vi "SHARP_2Y0A21_(SubVI).vi"(10 "Stop":bool, 11 "Calibration Parameters":cluster{"m":dbl, "b":dbl, "k":dbl, "c":dbl}={"m"=1.8233599662780762, "b"=0.2962961196899414, "k"=0.17500019073486328, "c"=0.17500019073486328}) -> (0 "error out":errorcluster, 2 "Gauge":dbl(knob) scale=10.0..150.0, 3 "Distance Waveform":dbl(graph))   [LabVIEW 2016]
uses:
  <vilib>/myRIO/Instrument Drivers/Onboard IO/AI/vis/Read.vi
  <vilib>/myRIO/Common/Instrument Driver Framework/myRIO v1.0/UART/vis/myRIO v1.0 Close UART.vi
  <vilib>/myRIO/Instrument Drivers/Onboard IO/AI/vis/Smart Open.vi
  <vilib>/Utility/error.llb/Error Cluster From Error Code.vi
  <vilib>/myRIO/Common/Instrument Driver Framework/myRIO v1.0/AI/vis/myRIO v1.0 Read AI.vi
  <vilib>/myRIO/Common/Instrument Driver Framework/Utilities/vis/FPGA Ref Manager.vi
  <vilib>/myRIO/Common/Instrument Driver Framework/myRIO v1.0/myRIO v1.0 Reset FPGA.vi
  <vilib>/myRIO/Common/Instrument Driver Framework/myRIO v1.0/IRQ/vis/myRIO v1.0 IRQ Info FGV.vi
  <vilib>/myRIO/Common/Instrument Driver Framework/myRIO v1.0/IRQ/vis/myRIO v1.0 Timer IRQ Info FGV.vi
  <vilib>/myRIO/Common/Instrument Driver Framework/myRIO v1.0/IRQ/vis/myRIO v1.0 ISR Agent.vi
  <vilib>/myRIO/Instrument Drivers/Utilities/Utilities.lvlib
panel:
  out "Numeric":dbl
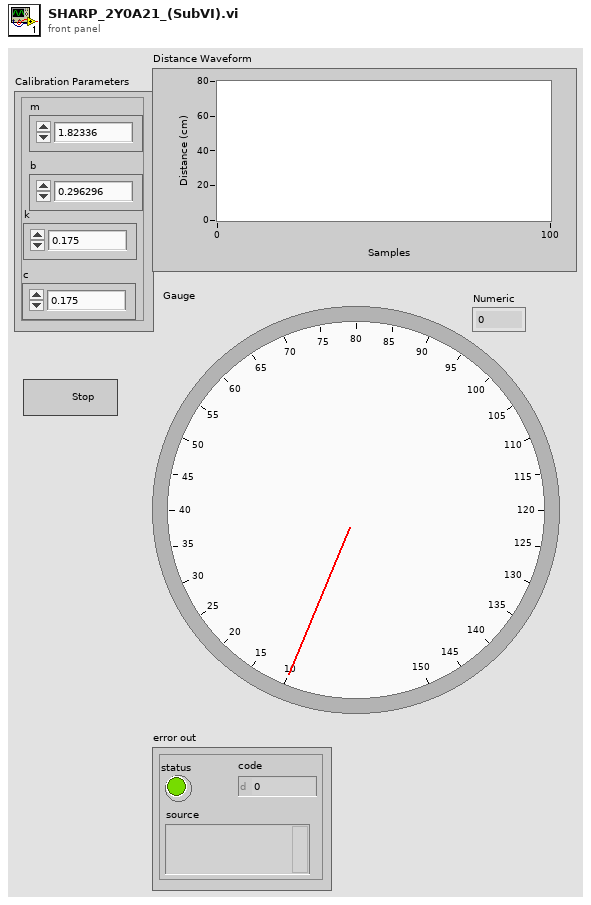
[diagram p1: front panel]
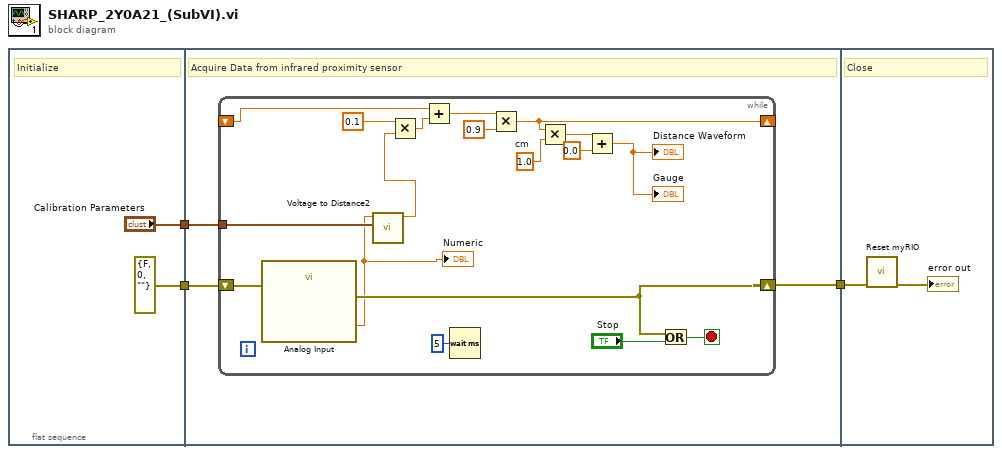
[diagram p0: block diagram]
diagram:
  n1 = flat-sequence {
    tunnel: ["Calibration Parameters"] -> w3
    tunnel: [errorcluster {"status"=FALSE, "code"=0, "source"=""} ("error out")] -> w2
    tunnel: w3 -> [w8]
    tunnel: w2 -> [w7]
    tunnel: [w6] -> w1
    tunnel: w1 -> [w28]
    frame #0 {
      # "Initialize"
    }
    frame #1 {
      # "Acquire Data from infrared proximity sensor"
      n2 = while {
        tunnel: w8 -> [w26]
        shift-right: [w21] -> w6
        shift-left: w7 -> [w22]
        shift-right: [w13] -> _
        shift-left: _ -> [w19]
        stop <- w24 stop-if-true
        w12 = 1.0  # cm
        n3 = call "Analog Input"("error in (no error)"=w22) -> ("A/AI0 (Pin 3)"=w9:dbl, "error out"=w21:errorcluster)  [unwired: 25 in]
        "Numeric" <- w9
        n4 = call "Voltage to Distance2.vi"("Voltage"=w9, "Calibration Parameters"=w26) -> ("Distance"=w10:dbl)  [unwired: 8 in]
        n5 = Multiply(x=0.1 ("y"), y=w10) -> (x*y=w17:dbl)
        n6 = Add(x=w19, y=w17) -> (x+y=w18:dbl)
        n7 = Wait (ms)(milliseconds to wait=u32 5) -> ()  [unwired: 1 out]
        n8 = Multiply(x=w18, y=0.9) -> (x*y=w13:dbl)
        n9 = Multiply(x=w13, y=w12) -> (x*y=w15:dbl)
        n10 = Add(x=w15, y=0.0) -> (x+y=→"Distance Waveform" →"Gauge":dbl)
        n11 = Or(x=w21, y="Stop") -> (x .or. y?=w24:bool)
      }
    }
    frame #2 {
      # "Close"
      n12 = call <vilib>:"Reset myRIO.vi"("error in (no error)"=w28) -> ("error out"=→"error out":errorcluster)  [unwired: 10 in]
    }
  }
